vi "StarWarsMelody.vi"() -> ()   [LabVIEW 2014]
panel:
  out "Array":dbl[][](array[numeric])
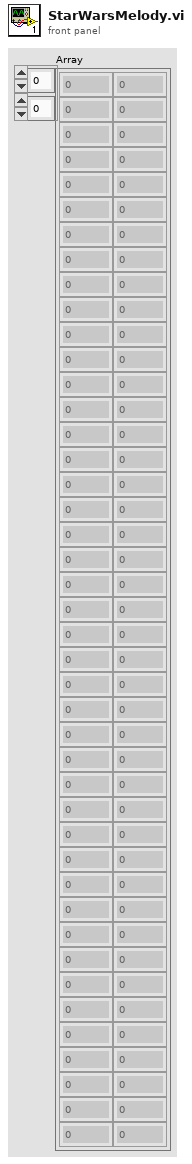
[diagram p1: front panel]
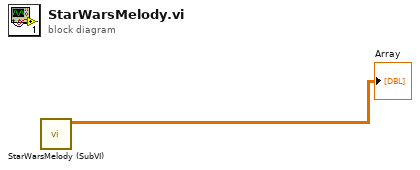
[diagram p0: block diagram]
diagram:
  n1 = call "StarWarsMelody (SubVI).vi"() -> ("Array"=→"Array":dbl[][])  [unwired: 11 in]
